vi "Write Refnum String.vi"(8 "error in (no error)":errorcluster, 10 "Refnum String":string, 11 "Arithmetic_Operations in":refnum<class "Arithmetic_Operations.lvclass">) -> (0 "error out":errorcluster, 3 "Arithmetic_Operations out":refnum<class "Arithmetic_Operations.lvclass">)   [LabVIEW 2020, in "Arithmetic_Operations.lvclass"]
uses:
  Arithmetic_Operations.lvclass
  Arithmetic_Operations.lvclass/Arithmetic_Operations.ctl
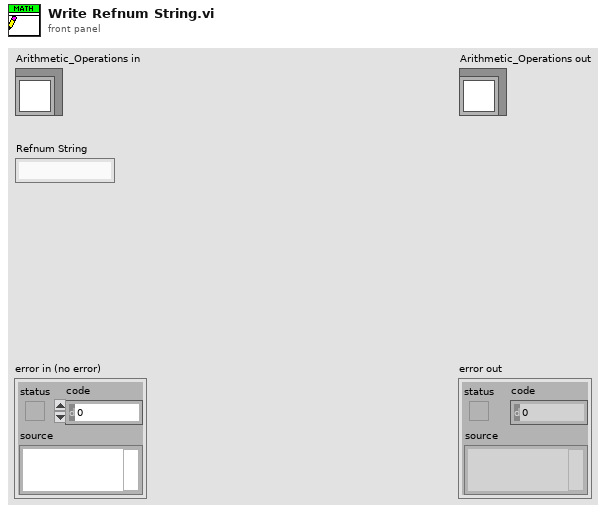
[diagram p1: front panel]
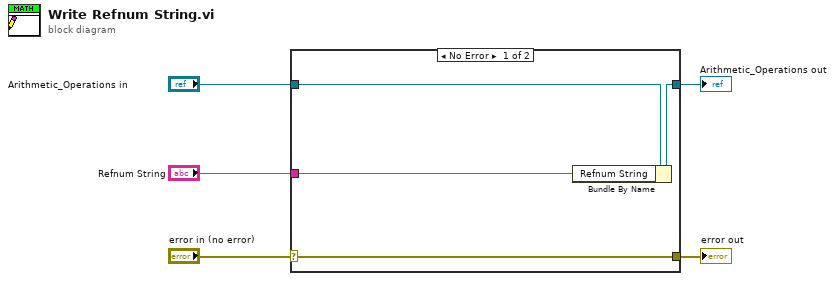
[diagram p0: block diagram]
diagram:
  n1 = case shown="No Error" "error in (no error)" {
    selector: "error in (no error)" -> [w9 w10]
    tunnel: [w9 w10] -> w4
    tunnel: [w7 w11] -> w2
    tunnel: "Arithmetic_Operations in" -> [w8 w11]
    tunnel: "Refnum String" -> [w6 _]
    frame No Error {
      n2 = Bundle By Name(cluster=w8, "Refnum String"=w6) -> (w7:refnum<class "Arithmetic_Operations.lvclass">)
    }
    frame Error {
    }
  }
  "error out" <- w4
  "Arithmetic_Operations out" <- w2
